vi "save_camera_images.vi"(4 "error in":errorcluster, 5 "frame_number":i32, 6 "Image":picture, 7 "Path to save image":path) -> (0 "error out":errorcluster)   [LabVIEW 2019, in "Lib_Simx.lvlib"]
doc: "Tool to help save images directly from the the camera sensor into your system."
uses:
  Lib_Simx.lvlib
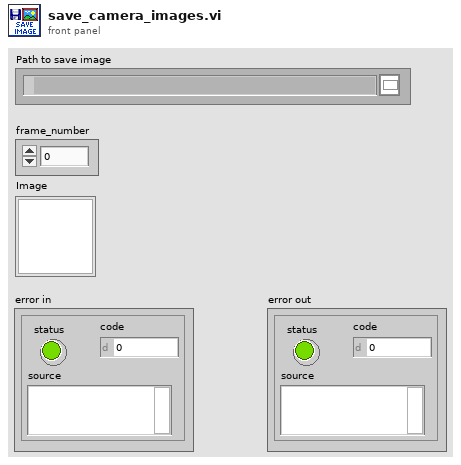
[diagram p1: front panel]
types:
  T1 = typedef "imagedata.ctl" = cluster{"image type":i32, "image depth":i32, "image":u8[], "mask":u8[], "colors":u32[], "Rectangle":cluster{"left":i16, "top":i16, "right":i16, "bottom":i16}}
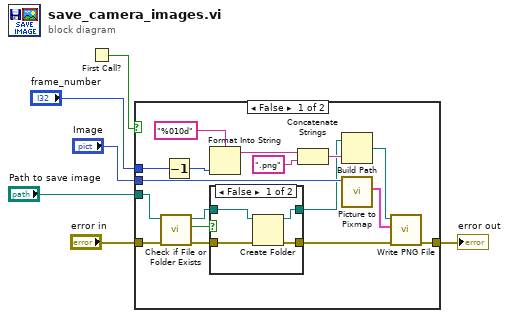
[diagram p0: block diagram]
diagram:
  n1 = First Call?() -> (First Call?: T/F=w1:bool)
  n2 = case shown="False" w1 {
    tunnel: [w22 w30] -> w6
    tunnel: "Path to save image" -> [w10 _]
    tunnel: "error in" -> [w12 w30]
    tunnel: "Image" -> [w18 _]
    tunnel: "frame_number" -> [w16 _]
    frame False {
      n3 = call <vilib>:"Check if File or Folder Exists.vi"("error in (no error)"=w12, "path"=w10) -> ("error out"=w13:errorcluster, "file or folder exists?"=w14:bool, "dup path"=w8:path)  [unwired: 7 in]
      n4 = Decrement(x=w16) -> (x-1=w7:i32)
      n5 = Format Into String(format string="%010d" ("initial string"), w7) -> (resulting string=w15:string)  [unwired: 2 in, 1 out]
      n6 = case shown="False" w14 {
        tunnel: w13 -> [w27 w29]
        tunnel: [w26 w29] -> w11
        tunnel: w8 -> [w25 w28]
        tunnel: [w24 w28] -> w9
        frame False {
          n7 = Create Folder(path (use dialog)=w25, error in=w27) -> (created path=w24:path, error out=w26:errorcluster)  [unwired: 1 in, 1 out]
        }
        frame True {
        }
      }
      n8 = Concatenate Strings(w15, ".png" ("string")) -> (w21:string)
      n9 = Build Path(base path=w9, name or relative path=w21) -> (appended path=w19:path)
      n10 = call <vilib>:"Picture to Pixmap.vi"("picture"=w18) -> ("image data"=w23:T1)  [unwired: 9 in, 1 out]
      n11 = call <vilib>:"Write PNG File.vi"("error in (no error)"=w11, "image data"=w23, "path to PNG file"=w19) -> ("error out"=w22:errorcluster)  [unwired: 7 in, 1 out]
    }
    frame True {
    }
  }
  "error out" <- w6
